vi "Z_HSw_BtnDown.vi"(8 "error in (no error)":errorcluster, 11 "Z_HSw_in":refnum<class "Z_HSw.lvclass">) -> (0 "error out":errorcluster, 2 "Data changed":bool, 3 "Z_HSw_out":refnum<class "Z_HSw.lvclass">)   [LabVIEW 2019, in "Z_HSw.lvclass"]
uses:
  Z_HSw.lvclass
  Z_HSw.lvclass/Z_HSw.ctl
  ctl/Z_HSw_state.ctl
  Z_source.ctl
  Timer Delay/Timers.lvlib
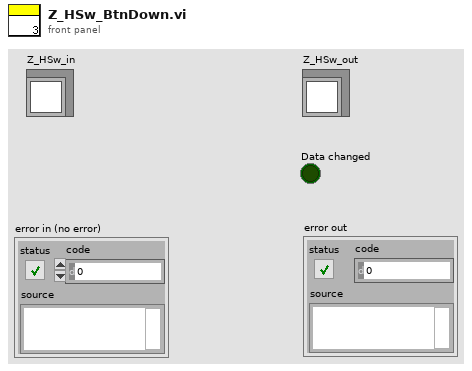
[diagram p1: front panel]
types:
  T1 = typedef "Z_HSw.lvclass/Z_HSw_state.ctl" = enum16{"init", "switch hand", "not hand", "hand", "switch auto", "not auto", "auto"}
  T2 = typedef "Z_source.ctl" = enum8{"initialize", "local disabled", "local hand", "hand", "auto", "dist"}
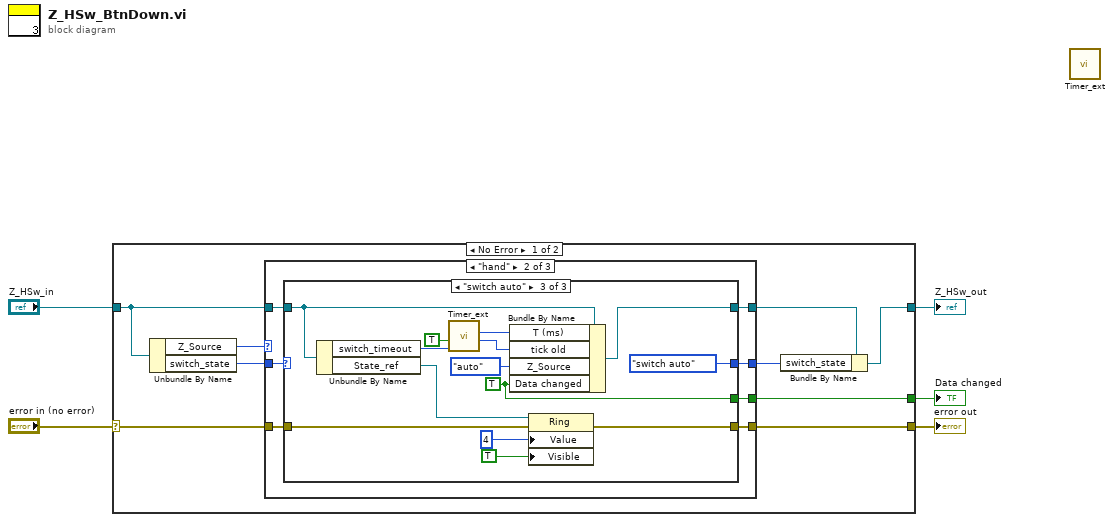
[diagram p0: block diagram]
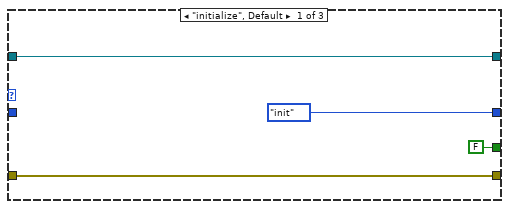
[diagram p2: hidden frame]
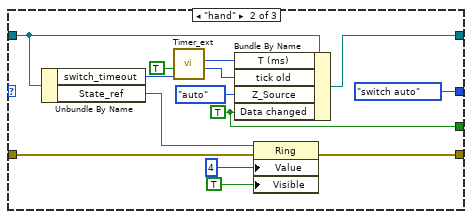
[diagram p4: hidden frame]
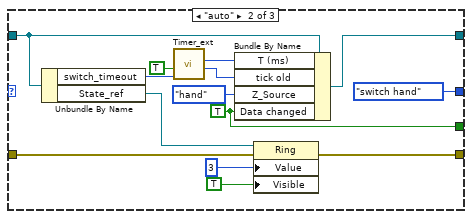
[diagram p6: hidden frame]
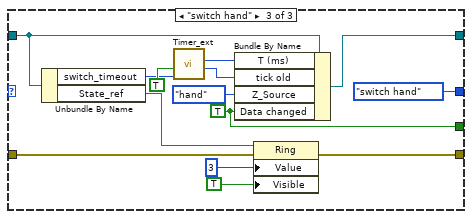
[diagram p7: hidden frame]
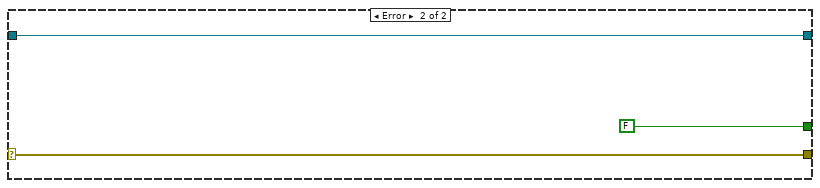
[diagram p8: hidden frame]
diagram:
  n1 = case shown="No Error" "error in (no error)" {
    selector: "error in (no error)" -> [w12 w97]
    tunnel: "Z_HSw_in" -> [w14 w96]
    tunnel: [w11 w97] -> w3
    tunnel: [w8 w96] -> w2
    tunnel: [w6 FALSE ("Data changed")] -> w1
    frame No Error {
      n2 = Unbundle By Name(w14) -> ("Z_Source"=w13:T2, "switch_state"=w10:T1)
      n3 = case shown="\"hand\"" w13 {
        tunnel: [Z_HSw_state."init" ("switch_state") w23 w61] -> w9
        tunnel: w14 -> [w18 w25 w62]
        tunnel: [w18 w21 w63] -> w7
        tunnel: w12 -> [w16 w22 w60]
        tunnel: [w16 w20 w59] -> w11
        tunnel: w10 -> [_ w24 w58]
        tunnel: [FALSE ("Data changed") w19 w57] -> w6
        frame "initialize", Default {
          # "local hand"
        }
        frame "hand" {
          # "local hand"
          n4 = case shown="\"switch auto\"" w24 {
            selector: w24 -> [w27 _ _]
            tunnel: [w28 w32 w46] -> w21
            tunnel: w25 -> [w28 w31 w45]
            tunnel: [w27 Z_HSw_state."switch auto" ("switch_state") Z_HSw_state."switch auto" ("switch_state")] -> w23
            tunnel: w22 -> [w26 w42 w56]
            tunnel: [w26 w41 w55] -> w20
            tunnel: [_ w29 w43] -> w19
            frame "init", Default {
            }
            frame "hand" {
              w29 = TRUE ("Data changed")
              n5 = Unbundle By Name(w31) -> ("switch_timeout"=w35:u32, "State_ref"=w38:refnum<vi>)
              n6 = call "Timer_ext.vi"("ms"=w35, "Load"=TRUE) -> ("tick"=w33:u32, "t ms"=w34:u32)  [unwired: 7 in, 1 out]
              n7 = Bundle By Name(cluster=w31, "T (ms)"=w34, "tick old"=w33, "Z_Source"=Z_source."auto", "Data changed"=w29) -> (w32:refnum<class "Z_HSw.lvclass">)
              n8 = property on="Property Node" class="Ring"(reference=w38, error in=w42, "Value"=u8 4 ("Z1_ind visu"), "Visible"=TRUE) -> (error out=w41:errorcluster)  [unwired: 1 out]
            }
            frame "switch auto" {
              w43 = TRUE ("Data changed")
              n9 = Unbundle By Name(w45) -> ("switch_timeout"=w49:u32, "State_ref"=w52:refnum<vi>)
              n10 = call "Timer_ext.vi"("ms"=w49, "Load"=TRUE) -> ("tick"=w47:u32, "t ms"=w48:u32)  [unwired: 7 in, 1 out]
              n11 = Bundle By Name(cluster=w45, "T (ms)"=w48, "tick old"=w47, "Z_Source"=Z_source."auto", "Data changed"=w43) -> (w46:refnum<class "Z_HSw.lvclass">)
              n12 = property on="Property Node" class="Ring"(reference=w52, error in=w56, "Value"=u8 4 ("Z1_ind visu"), "Visible"=TRUE) -> (error out=w55:errorcluster)  [unwired: 1 out]
            }
          }
        }
        frame "auto" {
          # "local hand"
          n13 = case shown="\"init\", Default" w58 {
            selector: w58 -> [w65 _ _]
            tunnel: [w66 w70 w84] -> w63
            tunnel: w62 -> [w66 w69 w83]
            tunnel: [w65 Z_HSw_state."switch hand" ("switch_state") Z_HSw_state."switch hand" ("switch_state")] -> w61
            tunnel: w60 -> [w64 w80 w94]
            tunnel: [w64 w79 w93] -> w59
            tunnel: [_ w67 w81] -> w57
            frame "init", Default {
            }
            frame "auto" {
              w67 = TRUE ("Data changed")
              n14 = Unbundle By Name(w69) -> ("switch_timeout"=w73:u32, "State_ref"=w76:refnum<vi>)
              n15 = call "Timer_ext.vi"("ms"=w73, "Load"=TRUE) -> ("tick"=w71:u32, "t ms"=w72:u32)  [unwired: 7 in, 1 out]
              n16 = Bundle By Name(cluster=w69, "T (ms)"=w72, "tick old"=w71, "Z_Source"=Z_source."hand", "Data changed"=w67) -> (w70:refnum<class "Z_HSw.lvclass">)
              n17 = property on="Property Node" class="Ring"(reference=w76, error in=w80, "Value"=u8 3 ("Z1_ind visu"), "Visible"=TRUE) -> (error out=w79:errorcluster)  [unwired: 1 out]
            }
            frame "switch hand" {
              w81 = TRUE ("Data changed")
              n18 = Unbundle By Name(w83) -> ("switch_timeout"=w87:u32, "State_ref"=w90:refnum<vi>)
              n19 = call "Timer_ext.vi"("ms"=w87, "Load"=TRUE) -> ("tick"=w85:u32, "t ms"=w86:u32)  [unwired: 7 in, 1 out]
              n20 = Bundle By Name(cluster=w83, "T (ms)"=w86, "tick old"=w85, "Z_Source"=Z_source."hand", "Data changed"=w81) -> (w84:refnum<class "Z_HSw.lvclass">)
              n21 = property on="Property Node" class="Ring"(reference=w90, error in=w94, "Value"=u8 3 ("Z1_ind visu"), "Visible"=TRUE) -> (error out=w93:errorcluster)  [unwired: 1 out]
            }
          }
        }
      }
      n22 = Bundle By Name(cluster=w7, "switch_state"=w9) -> (w8:refnum<class "Z_HSw.lvclass">)
    }
    frame Error {
    }
  }
  "Z_HSw_out" <- w2
  "error out" <- w3
  "Data changed" <- w1
  n23 = call "Timer_ext.vi"() -> ()  [unwired: 9 in, 3 out]
